vi "Not Equivalent Test 2.vi"() -> ()   [LabVIEW 2017]
uses:
  JSONtext.lvlib
  <vilib>/addons/_JKI Toolkits/Caraya/classes/Assert/Assert.lvclass
  <vilib>/addons/_JKI Toolkits/Caraya/classes/Test/Test.lvclass
panel:
  out "Equivalent":bool[](array[boolean])
  out "Not Equivalent":bool[](array[boolean])
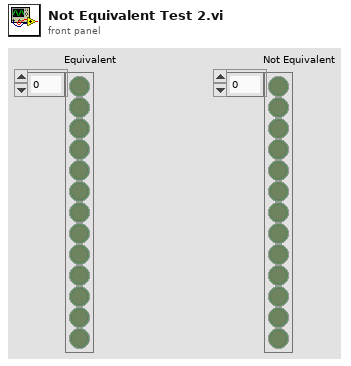
[diagram p1: front panel]
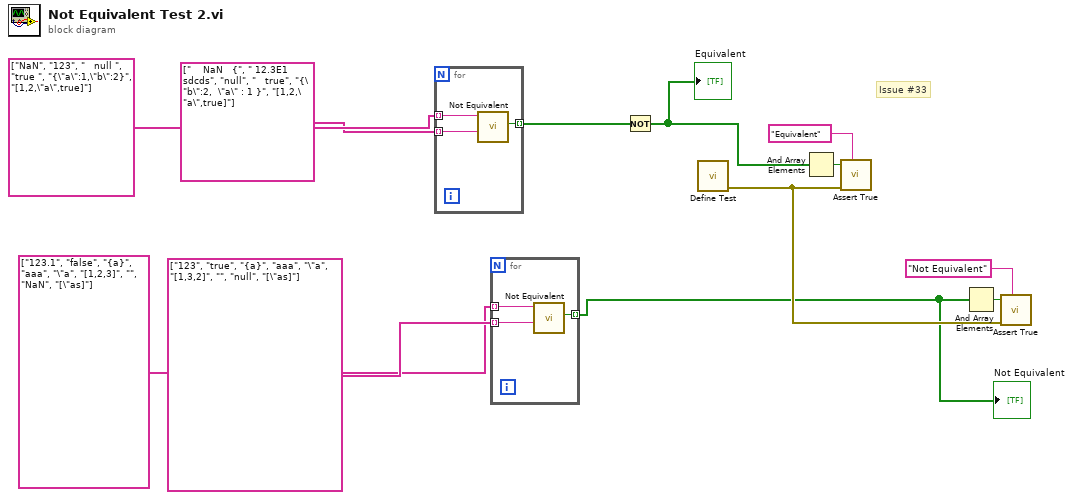
[diagram p0: block diagram]
diagram:
  # "Issue #33"
  n1 = for {
    tunnel: string[] ["NaN", "123", "   null ", "true ", "{\"a\":1,\"b\":2}", "[1,2,\"a\",true]"] ("JSON Object") -> [w15] mode=indexing
    tunnel: [w14] -> w2 mode=indexing
    tunnel: string[] ["    NaN   {", " 12.3E1   sdcds", "null", "   true", "{\"b\":2,  \"a\" : 1 }", "[1,2,\"a\",true]"] ("JSON Object") -> [w13] mode=indexing
    n2 = call "Not Equivalent.vi"("Other JSON"=w13, "JSON"=w15) -> ("Not Equivalent"=w14:bool)  [unwired: 8 in]
  }
  n3 = for {
    tunnel: string[] ["123.1", "false", "{a}", "aaa", "\"a", "[1,2,3]", "", "NaN", "[\"as]"] ("JSON Object") -> [w18] mode=indexing
    tunnel: [w17] -> w5 mode=indexing
    tunnel: string[] ["123", "true", "{a}", "aaa", "\"a", "[1,3,2]", "", "null", "[\"as]"] ("JSON Object") -> [w16] mode=indexing
    n4 = call "Not Equivalent.vi"("Other JSON"=w16, "JSON"=w18) -> ("Not Equivalent"=w17:bool)  [unwired: 8 in]
  }
  "Not Equivalent" <- w5
  n5 = Not(x=w2) -> (.not. x?=w1:bool[])
  "Equivalent" <- w1
  n6 = call <vilib>:"Define Test.vi"() -> ("error out"=w8:errorcluster)  [unwired: 11 in]
  n7 = And Array Elements(Boolean array=w1) -> (logical AND=w12:bool)
  n8 = call <vilib>:"Assert True.vi"("Label"="Equivalent", "error in (no error)"=w8, "True?"=w12) -> ()  [unwired: 8 in, 1 out]
  n9 = And Array Elements(Boolean array=w5) -> (logical AND=w9:bool)
  n10 = call <vilib>:"Assert True.vi"("Label"="Not Equivalent", "error in (no error)"=w8, "True?"=w9) -> ()  [unwired: 8 in, 1 out]
